vi "History Graph Message Loop.vi"(8 "error in (no error)":errorcluster, 11 "Message Queues":T1) -> (0 "error out":errorcluster)   [LabVIEW 2018, in "History Graph.lvlib"]
uses:
  History Graph.lvlib
  Main/Main Queue Cluster.ctl
  support/Message Queue/Message Cluster.ctl
  Controls/History Graph State Cluster.ctl
  d6897259-5d31-421a-b470-d285c4b10460.vi
  support/Message Queue/Enqueue Message (Single).vi
  support/Message Queue/Message Queue.lvlib
  Logging/Logging.lvlib
  support/User Event - Stop/User Event - Stop.lvlib
  TDMS Log/TDMS Log.lvlib
panel:
  out "Top Stop":timestamp
  in  "Exit Button":bool
  in  "Scrollbar":u64(c297)
  in  "Live Button":bool
  in  "Zoom Out Button":bool
  in  "Zoom In Button":bool
  out "Waveform Graph":waveform(dbl)[](graph)
  in  "Show Block Diagram":bool
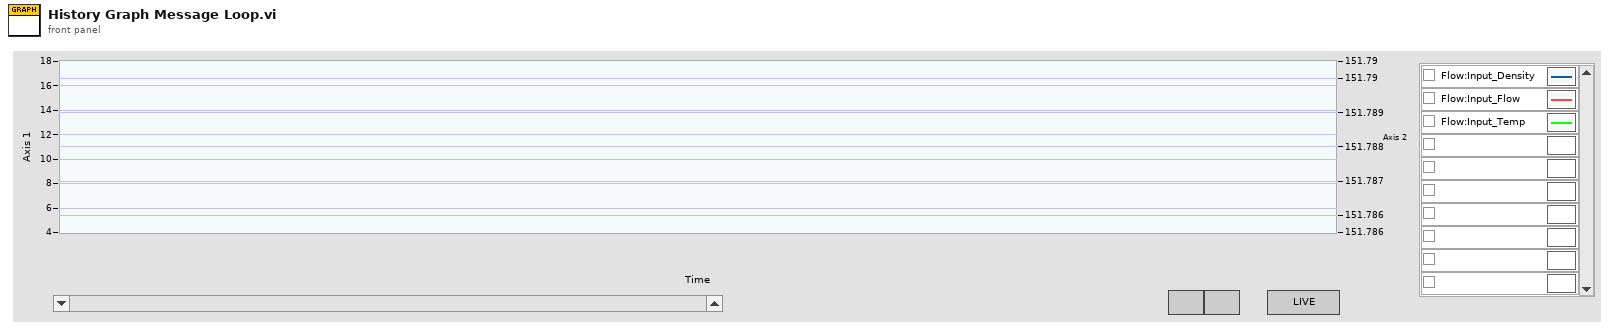
[diagram p1: front panel]
types:
  T1 = typedef "Main Queue Cluster.ctl" = cluster{"UI":refnum<queue>, "Waveform Loop":refnum<queue>, "CSV Log":refnum<queue>, "TDMS Log":refnum<queue>, "Graphs":refnum<queue>[], "DAQ":refnum<queue>, "Sequence":refnum<queue>, "TCP Write":refnum<queue>, "Sequence UI":refnum<queue>, "OPC UA Log":refnum<queue>, "TCP Read":refnum<queue>}
  T2 = typedef "History Graph.lvlib/History Graph State Cluster.ctl" = cluster{"Waveform Graph":refnum<vi>, "Graph Sample Period (ms)":i32, "Graph Data":waveform(dbl)[], "Graph Update Period (ms) 2":i32, "tdms file":refnum<k34>, "Num Samples in Window":i64}
  T3 = enum16{"open", "open or create", "create or replace", "create", "open (read-only)"}
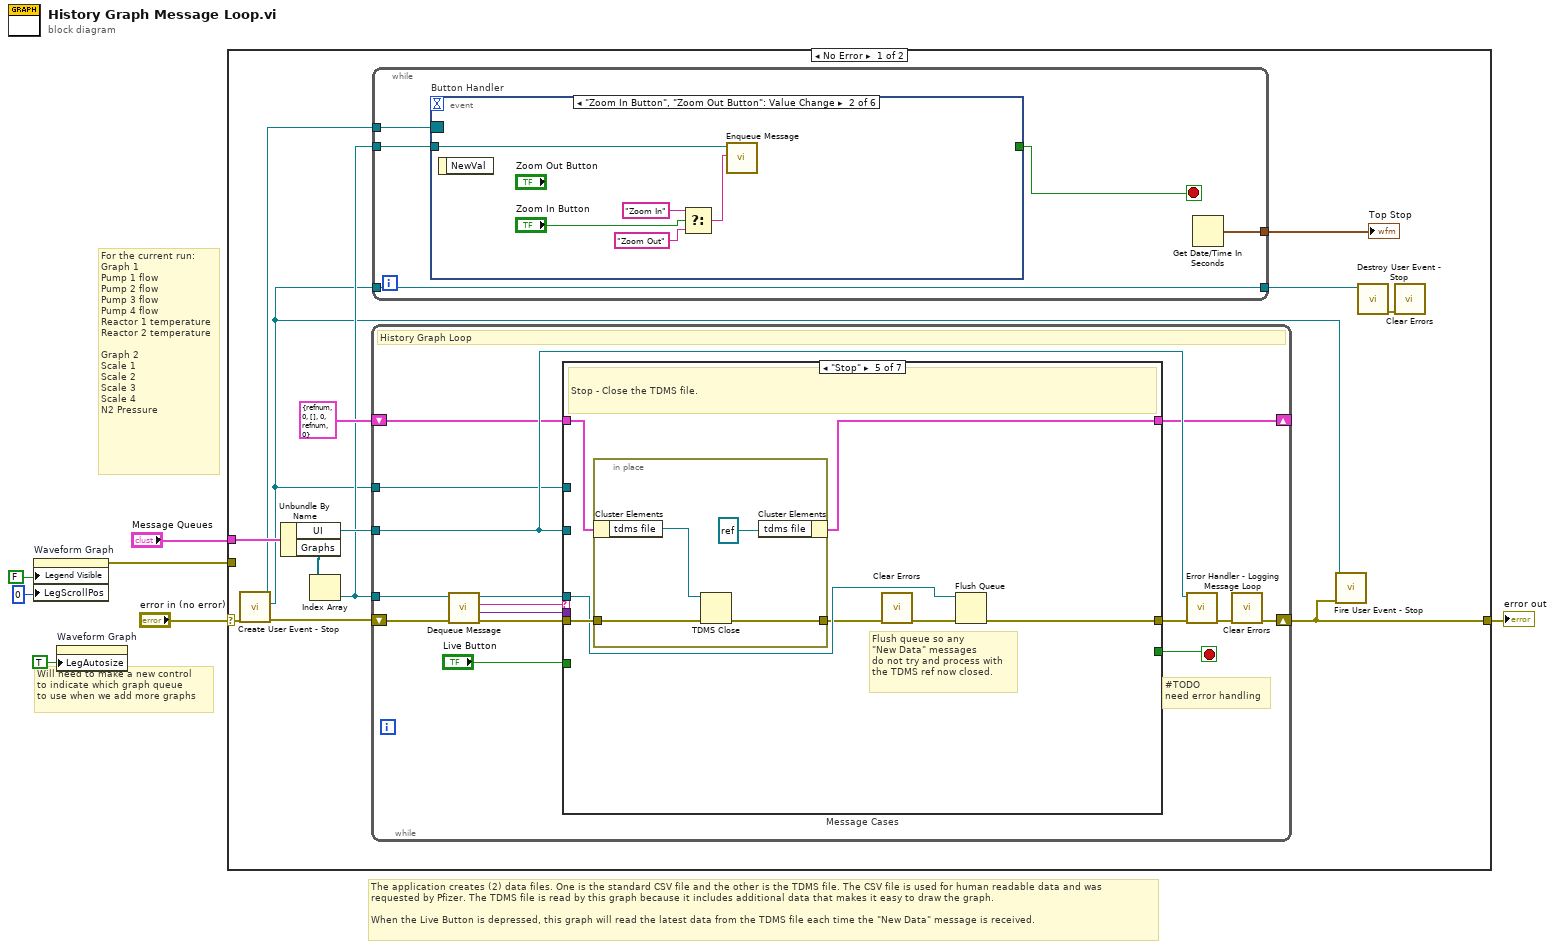
[diagram p0: block diagram]
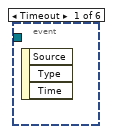
[diagram p2: hidden frame]
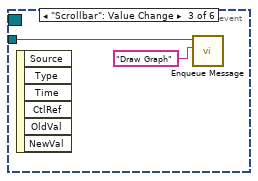
[diagram p3: hidden frame]
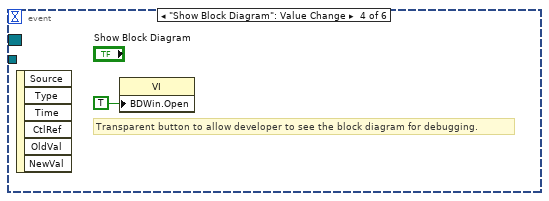
[diagram p4: hidden frame]
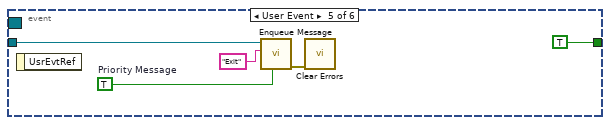
[diagram p5: hidden frame]
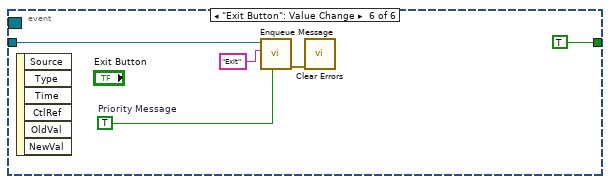
[diagram p6: hidden frame]
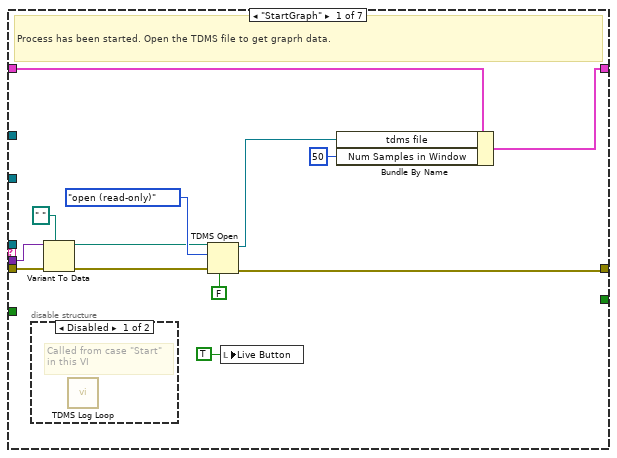
[diagram p7: hidden frame]
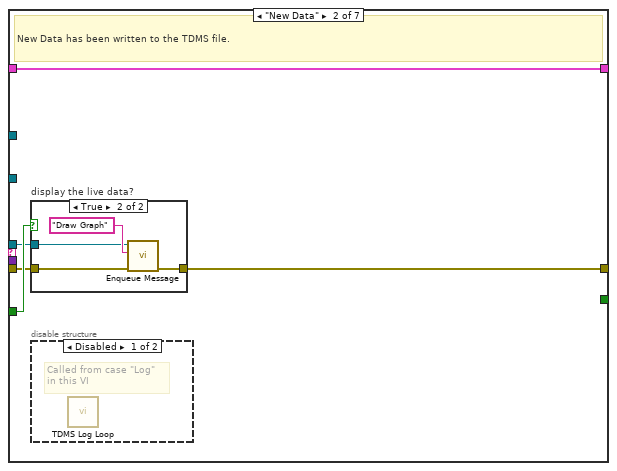
[diagram p9: hidden frame]
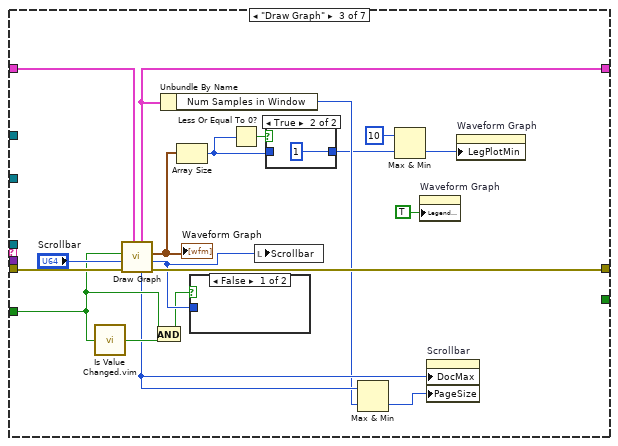
[diagram p12: hidden frame]
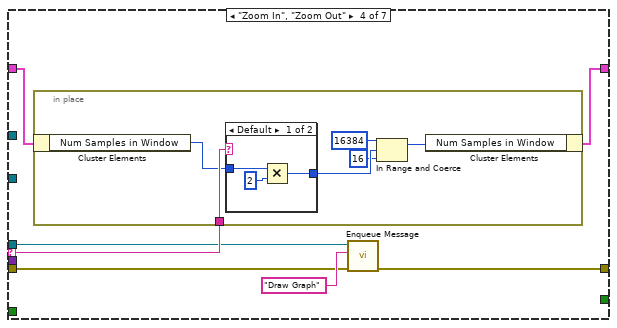
[diagram p15: hidden frame]
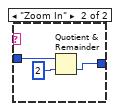
[diagram p16: hidden frame]
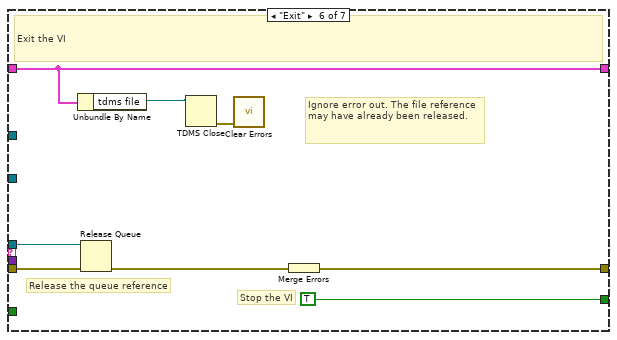
[diagram p17: hidden frame]
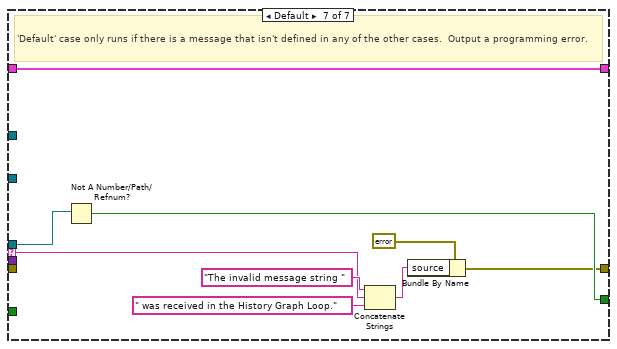
[diagram p18: hidden frame]
diagram:
  # "Will need to make a new control\nto indicate which graph queue\nto use when we add more graphs"
  # "The application creates (2) data files. One is the standard CSV file and the other is the TDMS file. The CSV file is used for human readable data and was\nrequested by Pfizer. The TDMS file is read by this graph because it includes additional data that makes it easy to draw the graph.\n\nWhen the Live Button is depressed, this graph will read the latest data from the TDMS file each time the \"New Data\" message is received."
  # "For the current run:\nGraph 1\nPump 1 flow\nPump 2 flow\nPump 3 flow\nPump 4 flow\nReactor 1 temperature\nReactor 2 temperature\n\nGraph 2\nScale 1\nScale 2\nScale 3\nScale 4\nN2 Pressure"
  n1 = property on="Waveform Graph" class="WFGraph (strict)"("Legend Visible"=FALSE ("Legend:Visible"), "LegScrollPos"=u32 0 ("Legend:Scroll Position")) -> (error out=w3:errorcluster)  [unwired: 2 in, 1 out]
  n2 = property on="Waveform Graph" class="WFGraph (strict)"("LegAutosize"=TRUE ("Legend:Autosize")) -> ()  [unwired: 2 in, 2 out]
  n3 = case shown="No Error" "error in (no error)" {
    selector: "error in (no error)" -> [w15 w150]
    tunnel: "Message Queues" -> [w20 _]
    tunnel: [w10 w150] -> w5
    tunnel: w3 -> [_ _]
    frame No Error {
      n4 = call "Create User Event - Stop.vi"("error in (no error)"=w15) -> ("error out"=w14:errorcluster, "User Event - Stop"=w9:refnum<user-event>, "Stop Event Registration Refnum"=w13:refnum<event-registration>)  [unwired: 8 in]
      n5 = Unbundle By Name(w20) -> ("UI"=w19:refnum<queue>, "Graphs"=w17:refnum<queue>[])
      n6 = Index Array(array=w17) -> (element=w16:refnum<queue>)  [unwired: 1 in]
      n7 = while {
        tunnel: w16 -> [w52]
        shift-right: [w49] -> _
        shift-left: T2 {"Waveform Graph"=refnum, "Graph Sample Period (ms)"=0, "Graph Data"=[], "Graph Update Period (ms) 2"=0, "tdms file"=refnum, "Num Samples in Window"=0} ("History Graph State") -> [w50]
        shift-right: [w45] -> w10
        shift-left: w14 -> [w57]
        tunnel: w19 -> [w51]
        tunnel: w9 -> [w47]
        stop <- w58 stop-if-true
        # "#TODO\nneed error handling"
        # "History Graph Loop"
        n8 = call "Dequeue Message.vi"("error in (no error)"=w57, "Message Queue"=w52) -> ("error out"=w56:errorcluster, "Message Data"=w54:variant, "Message"=w55:string, "dup Message Queue"=w53:refnum<queue>)  [unwired: 6 in]
        n9 = case "Message Cases" shown="\"Stop\"" w55 {
          selector: w55 -> [_ _ _ w109 _ _ w141]
          tunnel: w53 -> [_ w73 _ w108 w127 w137 w148]
          tunnel: w56 -> [w67 w74 w100 w105 w128 w138 _]
          tunnel: [w62 w72 w99 w106 w126 w139 w142] -> w44
          tunnel: w50 -> [w64 w76 w98 w104 w123 w135 w149]
          tunnel: [w61 w76 w92 w103 w122 w135 w149] -> w49
          tunnel: [_ _ _ _ _ TRUE w147] -> w58
          tunnel: w54 -> [w68 _ _ _ _ _ _]
          tunnel: w51 -> [_ _ _ _ _ _ _]
          tunnel: "Live Button" -> [_ w75 w93 _ _ _ _]
          tunnel: w47 -> [_ _ _ _ _ _ _]
          frame "StartGraph" {
            # "Process has been started. Open the TDMS file to get graprh data."
            n10 = disable-structure shown="Disabled" {
              frame Disabled {
                # "Called from case \"Start\"\nin this VI"
                n11 = call "TDMS Log Loop.vi"() -> ()  [unwired: 11 in, 1 out]
              }
              frame Enabled {
              }
            }
            n12 = Variant To Data(error in=w67, type=path " ", Variant=w68) -> (data=w66:path, error out=w65:errorcluster)
            n13 = TDMS Open(6:FALSE ("disable buffering (T)"), 8:w65, 10:T3."open (read-only)" ("operation"), 11:w66) -> (0:w62:errorcluster, 3:w63:refnum<k34>)  [unwired: 3 in]
            n14 = local write "Live Button"(TRUE ("Live Button")) -> ()
            n15 = Bundle By Name(cluster=w64, "tdms file"=w63, "Num Samples in Window"=i64 50) -> (w61:T2)
          }
          frame "New Data" {
            # "New Data has been written to the TDMS file."
            n16 = case "display the live data?" shown="True" w75 {
              tunnel: w74 -> [w77 w80]
              tunnel: w73 -> [_ w79]
              tunnel: [w77 w78] -> w72
              frame False {
              }
              frame True {
                n17 = call-poly "Enqueue Message.vi"("error in (no error)"=w80, "Message"="Draw Graph", "Message Queue"=w79) -> ("error out"=w78:errorcluster)  [unwired: 7 in, 1 out]
              }
            }
            n18 = disable-structure shown="Disabled" {
              frame Disabled {
                # "Called from case \"Log\"\nin this VI"
                n19 = call "TDMS Log Loop.vi"() -> ()  [unwired: 11 in, 1 out]
              }
              frame Enabled {
              }
            }
          }
          frame "Draw Graph" {
            n20 = call "Is Value Changed.vim"("value"=w93) -> ("changed or first call?"=w95:bool)
            n21 = call "Draw Graph.vi"("History Graph State in"=w98, "error in (no error)"=w100, "Scrollbar in"="Scrollbar", "Live Button"=w93) -> ("error out"=w99:errorcluster, "Scrollbar out"=w96:u64, "Waveform Graph"=w88:waveform(dbl)[], "Number of values in file"=w91:u64, "History Graph State out"=w92:T2)  [unwired: 3 in]
            "Waveform Graph" <- w88
            n22 = And(x=w93, y=w95) -> (x .and. y?=w94:bool)
            n23 = Unbundle By Name(w92) -> ("Num Samples in Window"=w90:i64)
            n24 = Array Size(array=w88) -> (size(s)=w82:i32)
            n25 = case shown="False" w94 {
              tunnel: w96 -> [_ _]
              frame False {
              }
              frame True {
              }
            }
            n26 = Less Or Equal To 0?(x=w82) -> (x <= 0?=w84:bool)
            n27 = local write "Scrollbar"(w96) -> ()
            n28 = case shown="True" w84 {
              tunnel: [w101 1] -> w83
              tunnel: w82 -> [w101 _]
              frame False {
              }
              frame True {
              }
            }
            n29 = Max & Min(x=w91, y=w90) -> (min(x,y)=w89:u64)  [unwired: 1 out]
            n30 = Max & Min(x=10, y=w83) -> (min(x,y)=w85:i32)  [unwired: 1 out]
            n31 = property on="Waveform Graph" class="WFGraph (strict)"("Legend Visible"=TRUE ("Legend:Visible")) -> ()  [unwired: 2 in, 2 out]
            n32 = property on="Scrollbar" class="Scroll (strict)"("DocMax"=w91, "PageSize"=w89) -> ()  [unwired: 2 in, 2 out]
            n33 = property on="Waveform Graph" class="WFGraph (strict)"("LegPlotMin"=w85) -> ()  [unwired: 2 in, 2 out]
          }
          frame "Zoom In", "Zoom Out" {
            n34 = in-place {
              in-place-border: w109 -> [w115]
              n35 = in-place-cluster #1(w104) -> ("Num Samples in Window"=w111:i64)
              n36 = case shown="Default" w115 {
                tunnel: w111 -> [w117 w120]
                tunnel: [w116 w119] -> w114
                frame Default {
                  n37 = Multiply(x=w117, y=i64 2) -> (x*y=w116:i64)
                }
                frame "Zoom In" {
                  n38 = Quotient & Remainder(x=w120, y=i64 2) -> (floor(x/y)=w119:i64)  [unwired: 1 out]
                }
              }
              n39 = In Range and Coerce(upper limit=i64 16384, x=w114, lower limit=i64 16) -> (coerced(x)=w110:i64)  [unwired: 1 out]
              n40 = in-place-cluster #1("Num Samples in Window"=w110) -> (w103:T2)
            }
            n41 = call-poly "Enqueue Message.vi"("error in (no error)"=w105, "Message"="Draw Graph", "Message Queue"=w108) -> ("error out"=w106:errorcluster)  [unwired: 7 in, 1 out]
          }
          frame "Stop" {
            # "Flush queue so any\n\"New Data\" messages \ndo not try and process with\nthe TDMS ref now closed."
            # "Stop - Close the TDMS file."
            n42 = in-place {
              in-place-border: w128 -> [w132]
              in-place-border: [w131] -> w125
              n43 = in-place-cluster #2(w123) -> ("tdms file"=w130:refnum<k34>)
              n44 = TDMS Close(8:w132, 11:w130) -> (0:w131:errorcluster)  [unwired: 1 out]
              n45 = in-place-cluster #2("tdms file"=refnum<k34> refnum) -> (w122:T2)
            }
            n46 = call <vilib>:"Clear Errors.vi"("error in (no error)"=w125) -> ("error out"=w124:errorcluster)  [unwired: 5 in, 1 out]
            n47 = Flush Queue(queue=w127, error in (no error)=w124) -> (error out=w126:errorcluster)  [unwired: 2 out]
          }
          frame "Exit" {
            # "Ignore error out. The file reference may have already been released."
            # "Release the queue reference"
            # "Stop the VI"
            # "Exit the VI"
            n48 = Unbundle By Name(w135) -> ("tdms file"=w134:refnum<k34>)
            n49 = Release Queue(queue=w137, error in (no error)=w138) -> (error out=w136:errorcluster)  [unwired: 1 in, 2 out]
            n50 = TDMS Close(11:w134) -> (0:w133:errorcluster)  [unwired: 1 in, 1 out]
            n51 = call <vilib>:"Clear Errors.vi"("error in (no error)"=w133) -> ()  [unwired: 5 in, 2 out]
            n52 = Merge Errors(w136) -> (w139:errorcluster)
          }
          frame Default {
            # "'Default' case only runs if there is a message that isn't defined in any of the other cases.  Output a programming error."
            n53 = Not A Number/Path/Refnum?(number/path/refnum=w148) -> (NaN/Path/Refnum?=w147:bool)
            n54 = Concatenate Strings("The invalid message string " ("string"), w141, " was received in the History Graph Loop." ("string")) -> (w143:string)
            n55 = Bundle By Name(cluster=errorcluster {"status"=TRUE, "code"=1, "source"=""} ("error constant"), "source"=w143) -> (w142:errorcluster)
          }
        }
        n56 = call "Error Handler - Logging Message Loop.vi"("error in (no error)"=w44, "Message Queue"=w51) -> ("dup error in"=w46:errorcluster)  [unwired: 8 in, 1 out]
        n57 = call <vilib>:"Clear Errors.vi"("error in (no error)"=w46) -> ("error out"=w45:errorcluster)  [unwired: 5 in, 1 out]
      }
      n58 = while {
        tunnel: w16 -> [w25]
        tunnel: w13 -> [w24]
        tunnel: [w22] -> w11
        tunnel: [w21] -> w8
        tunnel: w9 -> [w21]
        stop <- w23 stop-if-true
        n59 = event "Button Handler" shown="[1] \"Zoom In Button\", \"Zoom Out Button\": Value Change" {
          selector: w24 -> [_ _ _ _ _ _]
          dyn-events: _ -> [_ _ _ _ _ _]
          timeout: _ -> [_ _ _ _ _ _]
          tunnel: w25 -> [_ w30 w32 _ w38 w43]
          tunnel: [_ _ _ _ TRUE TRUE] -> w23
          event Timeout {
            n60 = event-data() -> ()  [unwired: 1 in, 3 out]
          }
          event "Zoom In Button", "Zoom Out Button": Value Change {
            n61 = event-data() -> ()  [unwired: 1 in, 1 out]
            n62 = Select(t="Zoom In" ("Message"), s="Zoom In Button", f="Zoom Out" ("Message")) -> (s? t:f=w26:string)
            n63 = call-poly "Enqueue Message.vi"("Message"=w26, "Message Queue"=w30) -> ()  [unwired: 8 in, 2 out]
          }
          event "Scrollbar": Value Change {
            n64 = event-data() -> ()  [unwired: 1 in, 6 out]
            n65 = call-poly "Enqueue Message.vi"("Message"="Draw Graph", "Message Queue"=w32) -> ()  [unwired: 8 in, 2 out]
          }
          event "Show Block Diagram": Value Change {
            # "Transparent button to allow developer to see the block diagram for debugging."
            n66 = event-data() -> ()  [unwired: 1 in, 6 out]
            n67 = property class="VI"("BDWin.Open"=TRUE ("Block Diagram Window:Open")) -> ()  [unwired: 2 in, 2 out]
          }
          event User Event {
            w35 = TRUE  # Priority Message
            n68 = event-data() -> ()  [unwired: 1 in, 1 out]
            n69 = call-poly "Enqueue Message.vi"("Priority Message? (F)"=w35, "Message"="Exit", "Message Queue"=w38) -> ("error out"=w34:errorcluster)  [unwired: 7 in, 1 out]
            n70 = call <vilib>:"Clear Errors.vi"("error in (no error)"=w34) -> ()  [unwired: 5 in, 2 out]
          }
          event "Exit Button": Value Change {
            w40 = TRUE  # Priority Message
            n71 = event-data() -> ()  [unwired: 1 in, 6 out]
            n72 = call-poly "Enqueue Message.vi"("Priority Message? (F)"=w40, "Message"="Exit", "Message Queue"=w43) -> ("error out"=w39:errorcluster)  [unwired: 7 in, 1 out]
            n73 = call <vilib>:"Clear Errors.vi"("error in (no error)"=w39) -> ()  [unwired: 5 in, 2 out]
          }
        }
        n74 = Get Date/Time In Seconds() -> (seconds since 1Jan1904=w22:timestamp)
      }
      "Top Stop" <- w11
      n75 = call "Fire User Event - Stop.vi"("error in (no error)"=w10, "User Event - Stop"=w9) -> ()  [unwired: 9 in, 1 out]
      n76 = call "Destroy User Event - Stop.vi"("User Event - Stop"=w8) -> ("error out"=w12:errorcluster)  [unwired: 10 in]
      n77 = call <vilib>:"Clear Errors.vi"("error in (no error)"=w12) -> ()  [unwired: 5 in, 2 out]
    }
    frame Error {
    }
  }
  "error out" <- w5
